vi "Open Google Campaign URL.vi"(4 "Campaign Content":string, 6 "Campaign Term":string, 7 "Campaign Medium":string, 8 "Error In":errorcluster, 9 "Campaign Source":string, 10 "Campaign Name":string, 11 "URL":string) -> (0 "Error Out":errorcluster, 3 "URL":string)   [LabVIEW 2020, in "LMH-Toolbox.lvlib"]
doc: "Build a google campaign URL and open in the default web browser."
uses:
  LMH-Toolbox.lvlib
  <vilib>/Platform/browser.llb/Open URL in Default Browser (string).vi
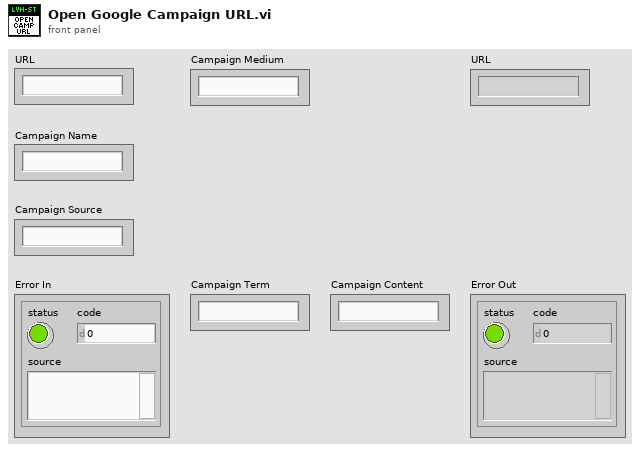
[diagram p1: front panel]
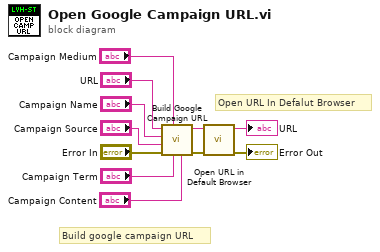
[diagram p0: block diagram]
diagram:
  # "Open URL In Defalut Browser"
  # "Build google campaign URL"
  n1 = call "Build Google Campaign URL.vi"("Campaign Content"="Campaign Content", "Campaign Term"="Campaign Term", "Campaign Medium"="Campaign Medium", "Error In"="Error In", "Campaign Source"="Campaign Source", "Campaign Name"="Campaign Name", "URL"="URL") -> ("Error Out"=w11:errorcluster, "Campaign URL"=w10:string)  [unwired: 3 in]
  n2 = call-poly <vilib>:"Open URL in Default Browser.vi"("error in (no error)"=w11, "URL"=w10) -> ("error out"=→"Error Out":errorcluster, "URL out"=→"URL":string)  [unwired: 4 in]
